vi "niFPGA BFGroup Twiddle Table 1024 U64.vi"(7 "address":fxp<+,10,10>) -> (4 "twid real":fxp<+/-,33,2> format="%.32g", 6 "twid imag":fxp<+/-,33,2> format="%.32g")   [LabVIEW 2017]
uses:
  <vilib>/Utility/error.llb/Clear Errors.vi
  <vilib>/rvi/Emulation/niFpgaSctlEmulationGetInTimedLoop.vi
  <vilib>/rvi/DataTransferAndStorage/Container/Common/niFpgaContainerGetUniqueNameForEmu.vi
  <vilib>/rvi/DataTransferAndStorage/Container/Common/niFpgaContainerSetEmuInfo.vi
  <vilib>/rvi/eio/common/nirviEmuReportErrorAndStop.vi
  <vilib>/rvi/Memory/Memory_Emulation/nirvimemoryEmulation.vi
  <vilib>/rvi/Memory/Memory_Emulation/nirvimemoryFastEmulation.vi
  <vilib>/rvi/Memory/Memory_Emulation/niFpgaMemoryEmulationCacheClearOnFirstRun.vi
  <vilib>/rvi/Memory/Memory_Emulation/nirvimemoryEmulationManagerCache_MakeExclusive.vi
  <vilib>/rvi/Memory/Memory_Emulation/niFpgaMemoryEmulationValidateCache.vi
  <vilib>/rvi/Memory/Memory_Emulation/nirvimemoryEmulationManagerCache_InsertValue.vi
  <vilib>/rvi/Memory/Memory_Emulation/nirvimemoryEmulationManagerCache_ReleaseExclusive.vi
  <vilib>/rvi/Memory/Memory_Emulation/nirvimemoryEmulationManagerCache_GetValue.vi
  <vilib>/rvi/Emulation/niFpgaEmulationIsFPGAContextNoSignature.vi
  <vilib>/rvi/Memory/Memory_Emulation/nirvimemoryEmulationManagerCache_SetValue.vi
  <vilib>/rvi/Emulation/niFpgaSctlEmulationResourceMgr.vi
  <vilib>/rvi/LocalResourceManager/LocalResourceManager.xnode
  <vilib>/rvi/DataTransferAndStorage/Container/XNode/niFpgaContainer.xnode
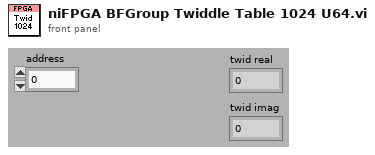
[diagram p1: front panel]
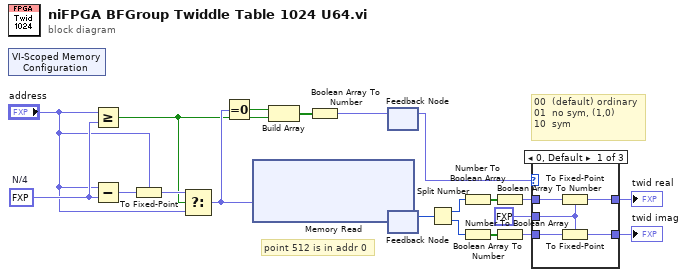
[diagram p0: block diagram]
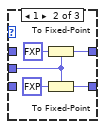
[diagram p2: hidden frame]
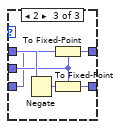
[diagram p3: hidden frame]
diagram:
  w15 = fxp<+,10,10> 512.0  # N/4
  # "point 512 is in addr 0"
  # "00  (default) ordinary\n01  no sym, (1,0)\n10  sym"
  n1 = xnode "VI-Scoped Memory Configuration"() -> ()  [unwired: 1 out]
  n2 = Greater Or Equal?(x="address", y=w15) -> (x >= y?=w1:bool)
  n3 = Subtract(x="address", y=w15) -> (x-y=w14:fxp<+/-,11,11>)
  n4 = To Fixed-Point(fixed-point type="address", number=w14) -> (fixed-point=w13:fxp<+,10,10>)
  n5 = Select(t=w13, s=w1, f="address") -> (s? t:f=w11:fxp<+,10,10>)
  n6 = Equal To 0?(x=w11) -> (x = 0?=w2:bool)
  n7 = xnode ("Memory Read")("Address"=w11) -> ("Data"=w21:u64)  [unwired: 2 out]
  n8 = Build Array(w2, w1) -> (w4:bool[])
  n9 = Boolean Array To Number(Boolean array=w4) -> (number=w3:fxp<+,2,2>)
  n10 = feedback-in #1(w3) -> ()
  n11 = feedback #1() -> (w5:fxp<+,2,2>)  [unwired: 1 out]
  n12 = feedback-in #2(w21) -> ()
  n13 = feedback #2() -> (w16:u64)  [unwired: 1 out]
  n14 = Split Number(x=w16) -> (hi(x)=w19:u32, lo(x)=w17:u32)
  n15 = Number To Boolean Array(number=w19) -> (Boolean array=w20:bool[])
  n16 = Number To Boolean Array(number=w17) -> (Boolean array=w18:bool[])
  n17 = Boolean Array To Number(Boolean array=w20) -> (number=w9:fxp<+/-,32,1>)
  n18 = Boolean Array To Number(Boolean array=w18) -> (number=w6:fxp<+/-,32,1>)
  n19 = case shown="0, Default" w5 {
    tunnel: w9 -> [w26 _ w36]
    tunnel: [w25 w30 w32] -> w8
    tunnel: w6 -> [w24 _ w33]
    tunnel: [w23 w28 w35] -> w7
    tunnel: fxp<+/-,33,2> 0.0 ("fixed-point type") -> [w22 w27 w34]
    frame 0, Default {
      n20 = To Fixed-Point(fixed-point type=w22, number=w26) -> (fixed-point=w25:fxp<+/-,33,2>)
      n21 = To Fixed-Point(fixed-point type=w22, number=w24) -> (fixed-point=w23:fxp<+/-,33,2>)
    }
    frame 1 {
      n22 = To Fixed-Point(fixed-point type=w27, number=fxp<+,1,1> 1.0 ("fixed-point type")) -> (fixed-point=w30:fxp<+/-,33,2>)
      n23 = To Fixed-Point(fixed-point type=w27, number=fxp<+,1,1> 0.0 ("fixed-point type")) -> (fixed-point=w28:fxp<+/-,33,2>)
    }
    frame 2 {
      n24 = Negate(x=w36) -> (-x=w37:fxp<+/-,33,2>)
      n25 = To Fixed-Point(fixed-point type=w34, number=w33) -> (fixed-point=w32:fxp<+/-,33,2>)
      n26 = To Fixed-Point(fixed-point type=w34, number=w37) -> (fixed-point=w35:fxp<+/-,33,2>)
    }
  }
  "twid real" <- w8
  "twid imag" <- w7
